vi "Obtain Tree Manager.vi"(8 "Error In":errorcluster) -> (0 "Error Out":errorcluster, 3 "Tree":T1)   [LabVIEW 2020, in "NI_VIAnCFGDataStructure.lvlib" / "Tree.lvclass"]
doc: "Obtain a reference to the Tree Manager. If this is the first reference initialize the Manager."
uses:
  <vilib>/addons/analyzer/VIAnCFGDataStructure/Tree Manager/Tree.lvclass
  <vilib>/addons/analyzer/VIAnCFGDataStructure/Tree Manager/Typedefs/Session Handle.ctl
  <vilib>/addons/analyzer/VIAnCFGDataStructure/Tree Manager/Tree.lvclass/Tree.ctl
  <vilib>/addons/analyzer/VIAnCFGDataStructure/Data Types/2D Bool/2D Bool.lvclass
  e:/builds/penguin/labview/branches/2020/dev/dist/vi.lib/addons/analyzer/VIAnCFGDataStructure/Tree Data/Tree Data.lvclass
  <vilib>/addons/analyzer/VIAnCFGDataStructure/Data Types/Bool Array/1D Bool.lvclass
  <vilib>/addons/analyzer/VIAnCFGDataStructure/Data Types/Bool/Bool.lvclass
  <vilib>/addons/analyzer/VIAnCFGDataStructure/Data Types/2D Flt/2D Flt.lvclass
  <vilib>/addons/analyzer/VIAnCFGDataStructure/Data Types/Flt Array/1D Flt.lvclass
  <vilib>/addons/analyzer/VIAnCFGDataStructure/Data Types/Float/Flt.lvclass
  <vilib>/addons/analyzer/VIAnCFGDataStructure/Data Types/2D Int/2D Int.lvclass
  <vilib>/addons/analyzer/VIAnCFGDataStructure/Data Types/Int Array/1D Int.lvclass
  <vilib>/addons/analyzer/VIAnCFGDataStructure/Data Types/Int/Int.lvclass
  <vilib>/addons/analyzer/VIAnCFGDataStructure/Data Types/2D Path/2D Path.lvclass
  <vilib>/addons/analyzer/VIAnCFGDataStructure/Data Types/Path Array/1D Path.lvclass
  <vilib>/addons/analyzer/VIAnCFGDataStructure/Data Types/Path/Path.lvclass
  <vilib>/addons/analyzer/VIAnCFGDataStructure/Data Types/2D String/2D String.lvclass
  <vilib>/addons/analyzer/VIAnCFGDataStructure/Data Types/String Array/1D String.lvclass
  <vilib>/addons/analyzer/VIAnCFGDataStructure/Data Types/String/String.lvclass
  <vilib>/Utility/LVClass/Get LV Class Name.vi
  <vilib>/addons/analyzer/VIAnCFGDataStructure/Tree Manager/Private/Make Short Class Name.vi
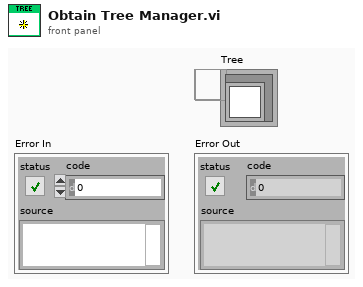
[diagram p1: front panel]
types:
  T1 = typedef "NI_VIAnCFGDataStructure.lvlib/Tree.lvclass/Session Handle.ctl" = refnum<data-value>
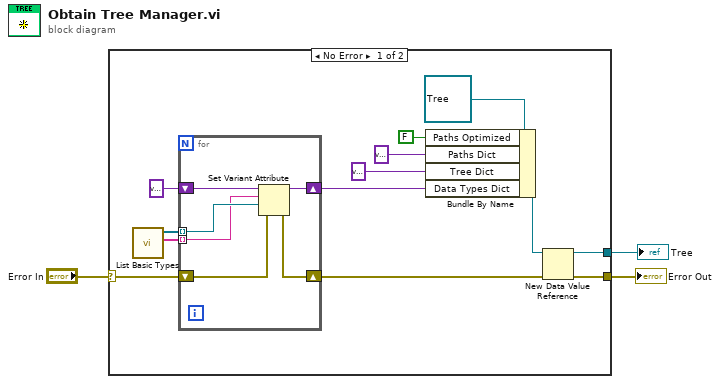
[diagram p0: block diagram]
diagram:
  n1 = case shown="No Error" "Error In" {
    selector: "Error In" -> [w11 w23]
    tunnel: [w7 w23] -> w2
    tunnel: [w8 _] -> w3
    frame No Error {
      n2 = call <vilib>:"List Basic Types.vi"() -> ("Long Class Names"=w4:string[], "Basic Types"=w12:refnum<class "Tree Data.lvclass">[])  [unwired: 9 in, 1 out]
      n3 = for {
        shift-right: [w21] -> w14
        shift-left: variant ("Tree Dictionary") -> [w22]
        tunnel: w12 -> [w20] mode=indexing
        shift-right: [w19] -> w10
        shift-left: w11 -> [w18]
        tunnel: w4 -> [w17] mode=indexing
        n4 = Set Variant Attribute(Variant=w22, name=w17, value=w20, error in=w18) -> (Variant out=w21:variant, error out=w19:errorcluster)  [unwired: 1 out]
      }
      n5 = Bundle By Name(cluster=refnum<class "Tree.lvclass"> refnum, "Paths Optimized"=FALSE, "Paths Dict"=variant ("Names Dict"), "Tree Dict"=variant ("Tree Dictionary"), "Data Types Dict"=w14) -> (w9:refnum<class "Tree.lvclass">)
      n6 = New Data Value Reference(data value=w9, error in=w10) -> (data value reference=w8:refnum<data-value>, error out=w7:errorcluster)
    }
    frame Error {
    }
  }
  "Tree" <- w3
  "Error Out" <- w2
